vi "svc_Find Greatest Common Divisor (DBL).vi"(9 "tolerance":dbl=1e-06, 10 "y":dbl=4947.0 format="%_8g", 11 "x":dbl=30.0 format="%_8g") -> (3 "gcd(x,y)":dbl=3.0 format="%_8g")   [LabVIEW 2017]
doc: "Finds the GCD of X and Y inputs."
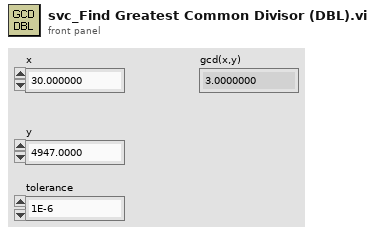
[diagram p1: front panel]
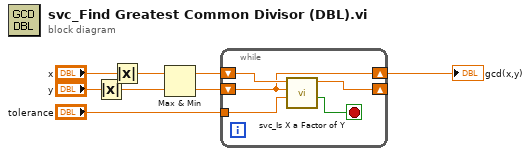
[diagram p0: block diagram]
diagram:
  n1 = Absolute Value(x="y") -> (abs(x)=w4:dbl)
  n2 = Absolute Value(x="x") -> (abs(x)=w5:dbl)
  n3 = Max & Min(x=w5, y=w4) -> (max(x,y)=w3:dbl, min(x,y)=w2:dbl)
  n4 = while {
    shift-right: [w12] -> _
    shift-left: w2 -> [w9]
    shift-right: [w9] -> w1
    shift-left: w3 -> [w10]
    tunnel: "tolerance" -> [w11]
    stop <- w13 stop-if-true
    n5 = call <vilib>:"svc_Is X a Factor of Y.vi"("tolerance"=w11, "X"=w9, "Y"=w10) -> ("divisible"=w13:bool, "residual"=w12:dbl)  [unwired: 6 in, 1 out]
  }
  "gcd(x,y)" <- w1
